vi "Obj_Detect.vi"(9 "Obj_Detect":bool, 10 "GPIO 1 Config":enum32{"Off", "Read", "Write", "PWM "}(radio), 11 "Speed_Main":dbl) -> (3 "Power_Detection":dbl)   [LabVIEW 2016, in "ArgoBotLib.lvlib"]
uses:
  ArgoBotLib.lvlib
panel:
  in  "DB":dbl=3.0
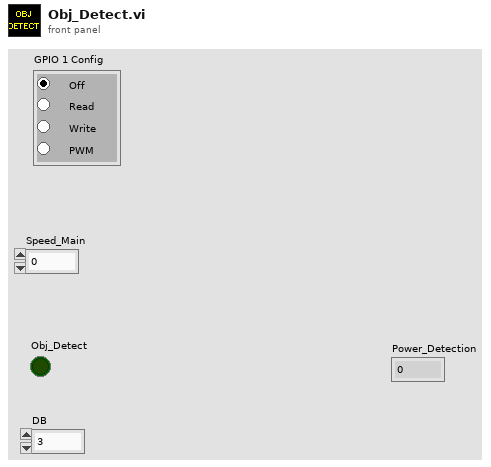
[diagram p1: front panel]
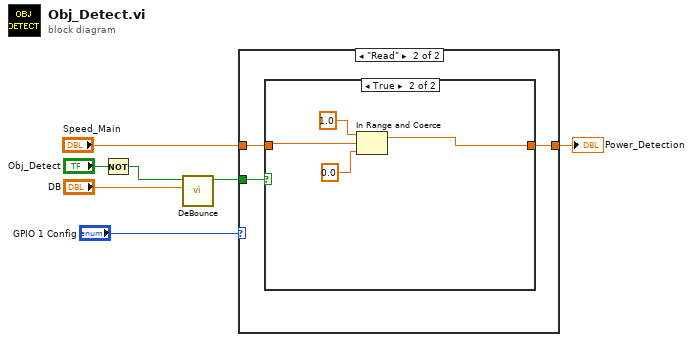
[diagram p0: block diagram]
diagram:
  n1 = Not(x="Obj_Detect") -> (.not. x?=w2:bool)
  n2 = call "DeBounce.vi"("DB_Count"="DB", "Value"=w2) -> ("BD_Value"=w6:bool)  [unwired: 9 in]
  n3 = case shown="\"Read\"" "GPIO 1 Config" {
    tunnel: w6 -> [_ w11]
    tunnel: "Speed_Main" -> [w8 w10]
    tunnel: [w8 w9] -> w4
    frame "Off", Default {
    }
    frame "Read" {
      n4 = case shown="True" w11 {
        tunnel: w10 -> [w12 w16]
        tunnel: [w12 w13] -> w9
        frame False {
        }
        frame True {
          n5 = In Range and Coerce(upper limit=1.0, x=w16, lower limit=0.0) -> (coerced(x)=w13:dbl)  [unwired: 1 out]
        }
      }
    }
  }
  "Power_Detection" <- w4
